vi "ExpEval_GetPrecedence.vi"(11 "Operator":string) -> (2 "Not found":bool, 3 "Precedence":i32)   [LabVIEW 2017, in "ExpressionEvaluator.lvlib"]
uses:
  <vilib>/addons/InsightCM/Utilities/ExpressionEvaluator/ExpressionEvaluator.lvlib
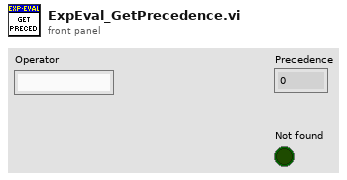
[diagram p1: front panel]
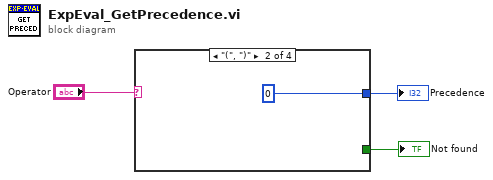
[diagram p0: block diagram]
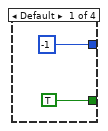
[diagram p2: hidden frame]
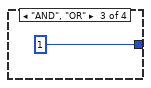
[diagram p3: hidden frame]
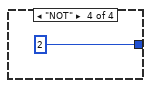
[diagram p4: hidden frame]
diagram:
  n1 = case shown="\"(\", \")\"" "Operator" {
    tunnel: [-1 0 1 2] -> w2
    tunnel: [TRUE _ _ _] -> w1
    frame Default {
    }
    frame "(", ")" {
    }
    frame "AND", "OR" {
    }
    frame "NOT" {
    }
  }
  "Precedence" <- w2
  "Not found" <- w1
